vi "Write Multiple Holding Registers1.vi"(7 "Unit_ID":T1, 8 "error in (no error)":errorcluster, 9 "holding register values":u16[](array[numeric]), 10 "starting address":u16, 11 "Modbus master in":refnum<class "TCP.lvclass">) -> (0 "error out":errorcluster, 3 "Modbus master out":refnum<class "TCP.lvclass">)   [LabVIEW 2019, in "NI_modbus_upd.lvlib"]
doc: "Writes values to contiguous holding registers. The maximum number of holding registers this VI can write is 123."
uses:
  NI_modbus_upd.lvlib
  TCP/TCP.lvclass
  Ctl/Unit_ID.ctl
  TCP/TCP.lvclass/TCP.ctl
  Function code mismatch error1.vi
  Error Generator1.vi
  Modbus Data Unit (PDU)/Construct PDU1.vi
  Utility/U16s to Bytes1.vi
  Read ADU Packet Master.vi
  Write ADU Packet Master.vi
  Modbus Data Unit (PDU)/Unflatten to PDU1.vi
  TCP/Protocol Read.vi
  TCP/Protocol Write.vi
  <vilib>/Utility/error.llb/Error Cluster From Error Code.vi
  Modbus Data Unit (PDU)/Deconstruct PDU1.vi
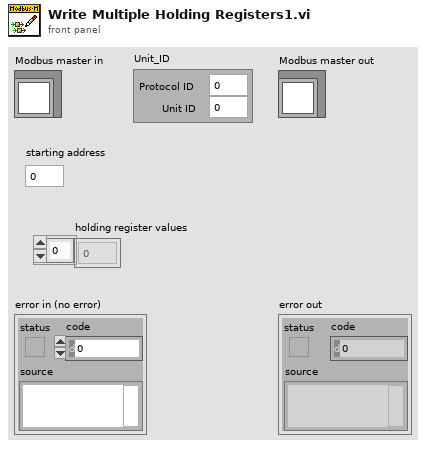
[diagram p1: front panel]
types:
  T1 = typedef "NI_modbus_upd.lvlib/Unit_ID.ctl" = cluster{"Protocol ID":u16, "Unit ID":u8}
  T2 = typedef "NI_modbus_upd.lvlib/MB Modbus Data Unit.ctl" = cluster{"function":T3, "Data":u8[]}
  T3 = typedef "NI_modbus_upd.lvlib/Function.ctl" = u8
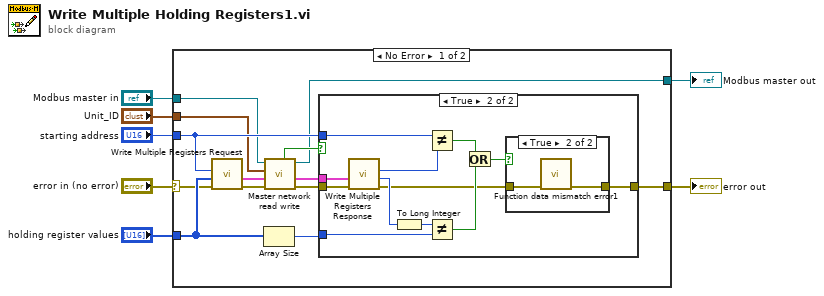
[diagram p0: block diagram]
diagram:
  n1 = case shown="No Error" "error in (no error)" {
    selector: "error in (no error)" -> [w8 w38]
    tunnel: "Modbus master in" -> [w11 w37]
    tunnel: [w19 w38] -> w4
    tunnel: [w13 w37] -> w5
    tunnel: "holding register values" -> [w16 _]
    tunnel: "starting address" -> [w18 _]
    tunnel: "Unit_ID" -> [w10 _]
    frame No Error {
      n2 = call "Write Multiple Registers Request.vi"("error in (no error)"=w8, "registers"=w16, "starting address"=w18) -> ("error out"=w20:errorcluster, "Modbus Data Unit out"=w9:T2)  [unwired: 7 in]
      n3 = Array Size(array=w16) -> (size(s)=w17:i32)
      n4 = call "Master network read write.vi"("error in (no error)"=w20, "Modbus Data Unit"=w9, "Unit_ID"=w10, "TCP in"=w11) -> ("error out"=w15:errorcluster, "Modbus data unit out"=w12:T2, "TCP out"=w13:refnum<class "TCP.lvclass">, "PDU valid?"=w14:bool)  [unwired: 4 in]
      n5 = case shown="True" w14 {
        tunnel: [w21 w30] -> w19
        tunnel: w18 -> [_ w24]
        tunnel: w17 -> [_ w28]
        tunnel: w15 -> [w21 w27]
        tunnel: w12 -> [_ w22]
        frame False {
        }
        frame True {
          n6 = call "Write Multiple Registers Response.vi"("error in (no error)"=w27, "Modbus Data Unit in"=w22) -> ("error out"=w26:errorcluster, "number of registers"=w29:u16, "start address"=w25:u16)  [unwired: 7 in]
          n7 = To Long Integer(number=w29) -> (32bit integer=w23:i32)
          n8 = Not Equal?(x=w24, y=w25) -> (x != y?=w32:bool)
          n9 = Not Equal?(x=w23, y=w28) -> (x != y?=w31:bool)
          n10 = Or(x=w32, y=w31) -> (x .or. y?=w33:bool)
          n11 = case shown="True" w33 {
            tunnel: [w34 w36] -> w30
            tunnel: w26 -> [w34 w35]
            frame False {
            }
            frame True {
              n12 = call "Function data mismatch error1.vi"("error in (no error)"=w35) -> ("error out"=w36:errorcluster)  [unwired: 10 in]
            }
          }
        }
      }
    }
    frame Error {
    }
  }
  "error out" <- w4
  "Modbus master out" <- w5
